vi "readHeaders.vi"(11 "HeaderRef In":refnum<data-value>) -> (3 "Headers":cluster{"key":string, "value":string}[](array[cluster]))   [LabVIEW 2020, in "net-http-client.lvclass"]
uses:
  net-http-client.lvclass
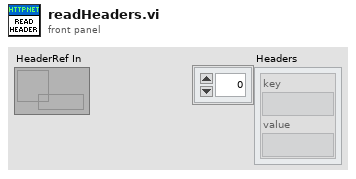
[diagram p1: front panel]
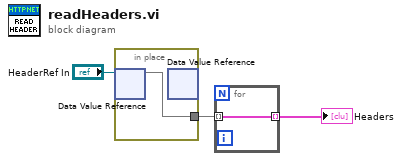
[diagram p0: block diagram]
diagram:
  n1 = in-place {
    in-place-border: [w4] -> w2
    n2 = in-place-dvr #1("HeaderRef In") -> (w4:map{string, string})  [unwired: 1 out]
    n3 = in-place-dvr #1() -> ()  [unwired: 1 in, 2 out]
  }
  n4 = for {
    tunnel: w2 -> [w5] mode=indexing
    tunnel: [w5] -> w3 mode=indexing
  }
  "Headers" <- w3
